vi "Gear_Rail.vi"() -> ()   [LabVIEW 2016]
uses:
  <vilib>/Rock Robotics/WPI/MotorControl/WPI_MotorControlDeviceRef.ctl
  <vilib>/Rock Robotics/WPI/MotorControl/WPI_MotorControlType.ctl
  <vilib>/Rock Robotics/SystemInterfaces/DIO/FPGA_DIOPWMChannel.ctl
  <vilib>/Rock Robotics/WPI/PWM/WPI_PWMDeadband.ctl
panel:
  in  "Potentiometer_Input":dbl
  in  "MotorControlDevRef":T1={"DeviceStatus"={"status"=FALSE, "code"=0, "source"=""}, "Type"=enum."PWM", "PWM"={"PWM Channel"=enum."Invalid", "DeadBand"={"Name"="", "maxPositivePwm"=0, "minPositivePwm"=0, "centerPwm"=0, "maxNegativePwm"=0, "minNegativePwm"=0, "angularRange"=0}}, "CAN"={"Device Number"=0, "SetOutput VI Ref"=variant(refnum<vi> refnum), "GetOutput VI Ref"=variant(refnum<vi> refnum), "Enable VI Ref"=variant(refnum<vi> refnum), "Disable VI Ref"=variant(refnum<vi> refnum), "Data"=variant}, "Invert"=FALSE}
  in  "Invert?":bool
  in  "Left_Button_Pressed?":bool
  in  "Right_Button_Pressed?":bool
  in  "Potentiometer_WantedPos":dbl
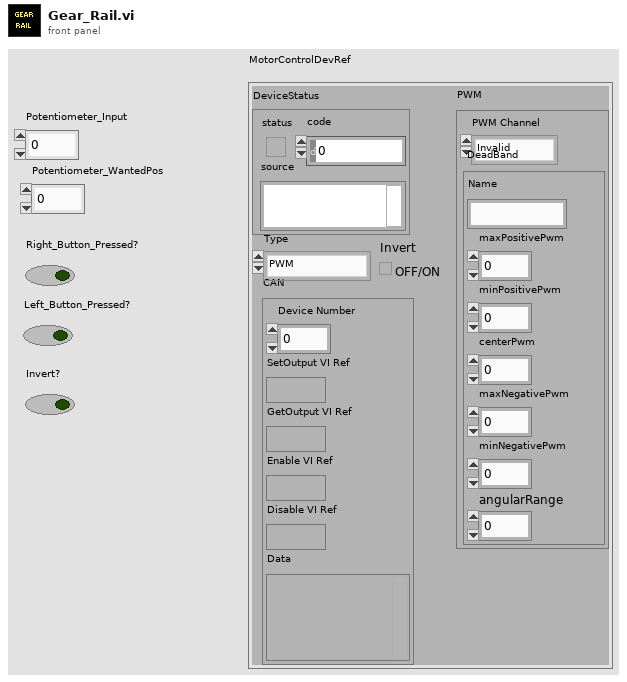
[diagram p1: front panel]
types:
  T1 = typedef "WPI_MotorControlDeviceRef.ctl" = cluster{"DeviceStatus":errorcluster, "Type":T2, "PWM":cluster{"PWM Channel":T3, "DeadBand":T4}, "CAN":cluster{"Device Number":u8, "SetOutput VI Ref":variant, "GetOutput VI Ref":variant, "Enable VI Ref":variant, "Disable VI Ref":variant, "Data":variant}, "Invert":bool}
  T2 = typedef "WPI_MotorControlType.ctl" = enum16{"PWM", "CAN"}
  T3 = typedef "FPGA_DIOPWMChannel.ctl" = enum8{"PWM 0", "PWM 1", "PWM 2", "PWM 3", "PWM 4", "PWM 5", "PWM 6", "PWM 7", "PWM 8", "PWM 9", "PWM MXP 0", "PWM MXP 1", "PWM MXP 2", "PWM MXP 3", "PWM MXP 4", "PWM MXP 5", "PWM MXP 6", "PWM MXP 7", "PWM MXP 8", "PWM MXP 9", "Invalid"}
  T4 = typedef "WPI_PWMDeadband.ctl" = cluster{"Name":string, "maxPositivePwm":i32, "minPositivePwm":i32, "centerPwm":i32, "maxNegativePwm":i32, "minNegativePwm":i32, "angularRange":u16}
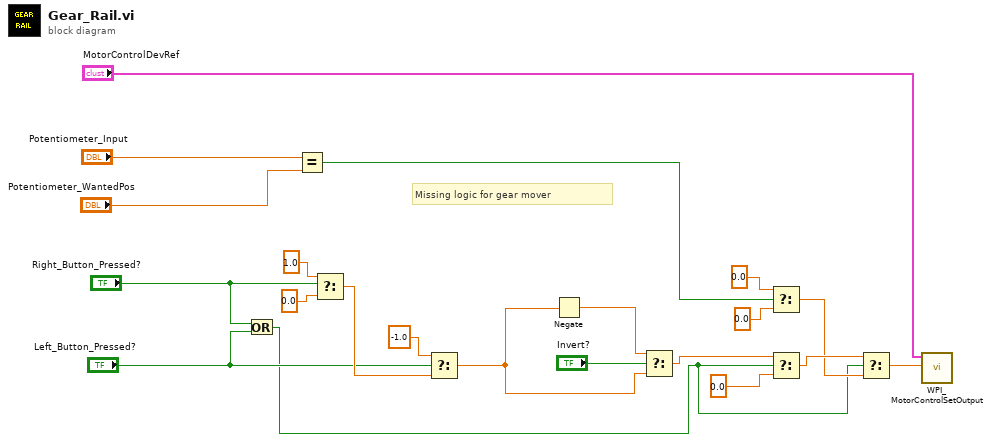
[diagram p0: block diagram]
diagram:
  # "Missing logic for gear mover"
  n1 = Or(x="Right_Button_Pressed?", y="Left_Button_Pressed?") -> (x .or. y?=w1:bool)
  n2 = Equal?(x="Potentiometer_Input", y="Potentiometer_WantedPos") -> (x = y?=w7:bool)
  n3 = Select(t=1.0, s="Right_Button_Pressed?", f=0.0) -> (s? t:f=w21:dbl)
  n4 = Select(t=-1.0, s="Left_Button_Pressed?", f=w21) -> (s? t:f=w19:dbl)
  n5 = Negate(x=w19) -> (-x=w18:dbl)
  n6 = Select(t=w18, s="Invert?", f=w19) -> (s? t:f=w9:dbl)
  n7 = Select(t=0.0, s=w7, f=0.0) -> (s? t:f=w2:dbl)
  n8 = Select(t=w9, s=w1, f=0.0) -> (s? t:f=w3:dbl)
  n9 = Select(t=w3, s=w1, f=w2) -> (s? t:f=w6:dbl)
  n10 = call <vilib>:"WPI_MotorControlSetOutput.vi"("Output"=w6, "MotorControlDevRef"="MotorControlDevRef") -> ()  [unwired: 7 in, 3 out]
